vi "CPP_AeroProbePtByPt.vi"(4 "Temperature (K)":dbl, 5 "Old5HoleProbe?":bool, 6 "Pressure (torr)":dbl, 7 "Data":dbl[][](array[numeric]), 9 "Zeroes":dbl[](array[numeric]), 10 "Calibration Folder Path":path) -> (1 "ExcessiveConeFraction":dbl, 2 "ValidFraction":dbl, 3 "VmagUVWCone":dbl[][](array[numeric]))   [LabVIEW 2013]
panel:
  in  "Graphs":bool
  in  "MaxCone":dbl=58.0
  out "Progress":dbl(slide) max=820.0 scale=-1.0..820.0
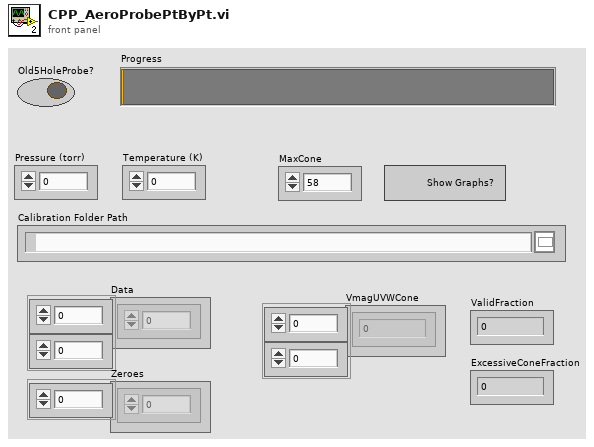
[diagram p1: front panel]
types:
  T1 = cluster{"[0]":dbl, "[1]":dbl, "[2]":dbl, "[3]":dbl, "[4]":dbl}
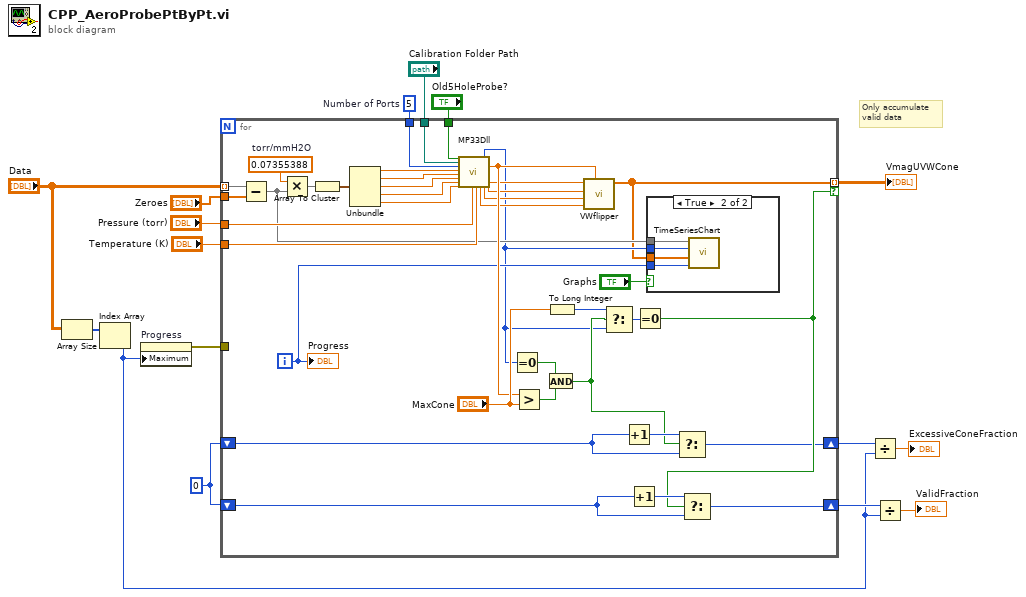
[diagram p0: block diagram]
diagram:
  w2 = 0
  w13 = 5  # Number of Ports
  # "Only accumulate\nvalid data"
  n1 = Array Size(array="Data") -> (size(s)=w6:i32[])
  n2 = Index Array(array=w6) -> (element=w3:i32)  [unwired: 1 in]
  n3 = property on="Progress" class="Slide (strict)"("Maximum"=w3) -> (error out=w9:errorcluster)  [unwired: 2 in, 1 out]
  n4 = for {
    tunnel: "Data" -> [w46] mode=indexing
    tunnel: "Zeroes" -> [w45]
    tunnel: [w18] -> w11 mode=indexing if=w31
    shift-right: [w44] -> w7
    shift-left: w2 -> [w37]
    tunnel: "Calibration Folder Path" -> [w43]
    tunnel: w13 -> [w42]
    tunnel: "Old5HoleProbe?" -> [w41]
    tunnel: "Temperature (K)" -> [w40]
    tunnel: "Pressure (torr)" -> [w39]
    tunnel: w9 -> [_]
    shift-right: [w28] -> w4
    shift-left: w2 -> [w30]
    i -> [w21]
    w54 = 0.07355388  # torr/mmH2O
    n5 = Subtract(x=w46, y=w45) -> (x-y=w20:dbl[])
    n6 = Multiply(x=w54, y=w20) -> (x*y=w53:dbl[])
    n7 = Array To Cluster(array=w53) -> (cluster=w52:T1)
    n8 = Unbundle(w52) -> ("[0]"=w51:dbl, "[1]"=w50:dbl, "[2]"=w49:dbl, "[3]"=w48:dbl, "[4]"=w47:dbl)
    n9 = call "MP33Dll.vi"("Old5HoleProbe?"=w41, "Calibration Folder Path"=w43, "Number of Ports"=w42, "P1 Torr"=w51, "P2 Torr"=w50, "P3 Torr"=w49, "P4 Torr"=w48, "P5 Torr"=w47, "Pref Torr"=w39, "TTot Kelvin"=w40) -> ("w m/s"=w22:dbl, "return type"=w19:i32, "v m/s"=w23:dbl, "Theta Degree"=w26:dbl, "VMagn m/s"=w25:dbl, "u  m/s"=w24:dbl)  [unwired: 7 in, 5 out]
    n10 = Equal To 0?(x=w19) -> (x = 0?=w35:bool)
    n11 = Greater?(x=w26, y="MaxCone") -> (0:w34:bool)
    n12 = And(x=w35, y=w34) -> (x .and. y?=w27:bool)
    n13 = To Long Integer(number="MaxCone") -> (32bit integer=w32:i32)
    n14 = call "VWflipper.vi"("Theta Degree"=w26, "Probe w m/s"=w22, "Probe v m/s"=w23, "Probe u  m/s"=w24, "VMagn m/s"=w25) -> ("VmagUVWCone"=w18:dbl[])  [unwired: 6 in]
    n15 = Select(t=w32, s=w27, f=w19) -> (s? t:f=w36:i32)
    n16 = Increment(x=w30) -> (x+1=w29:i32)
    n17 = Increment(x=w37) -> (x+1=w38:i32)
    n18 = Equal To 0?(x=w36) -> (x = 0?=w31:bool)
    n19 = case shown="True" "Graphs" {
      tunnel: w21 -> [_ w58]
      tunnel: w20 -> [_ w57]
      tunnel: w19 -> [_ w56]
      tunnel: w18 -> [_ w55]
      frame False {
      }
      frame True {
        n20 = call "TimeSeriesChart.vi"("iStep"=w58, "VmagUVWCone"=w55, "ReturnType"=w56, "netPressures"=w57) -> ()  [unwired: 8 in]
      }
    }
    n21 = Select(t=w29, s=w27, f=w30) -> (s? t:f=w28:i32)
    n22 = Select(t=w38, s=w31, f=w37) -> (s? t:f=w44:i32)
    "Progress" <- w21
  }
  "VmagUVWCone" <- w11
  n23 = Divide(x=w4, y=w3) -> (x/y=→"ExcessiveConeFraction":dbl)
  n24 = Divide(x=w7, y=w3) -> (x/y=→"ValidFraction":dbl)
